vi "notasdealumnos.vi"() -> ()   [LabVIEW 2013]
panel:
  out "Sobresaliente":bool
  out "Muy bueno":bool
  out "Bueno":bool
  out "Reprobado":bool
  out "91-100 Sobresaliente":dbl
  out "81-90 Muy bueno":dbl
  out "60-80 Bueno":dbl
  out "1-59 Reprobado":dbl
  out "Notas":dbl
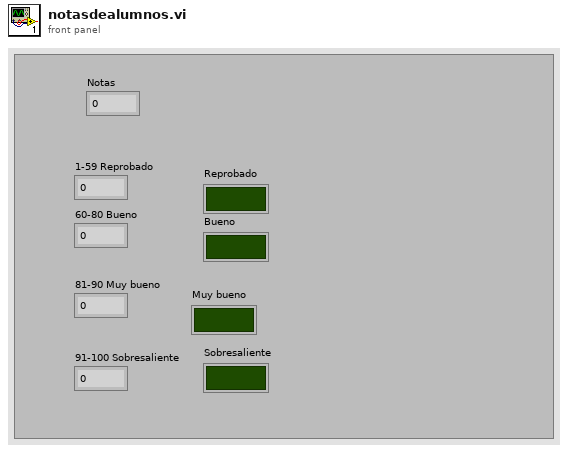
[diagram p1: front panel]
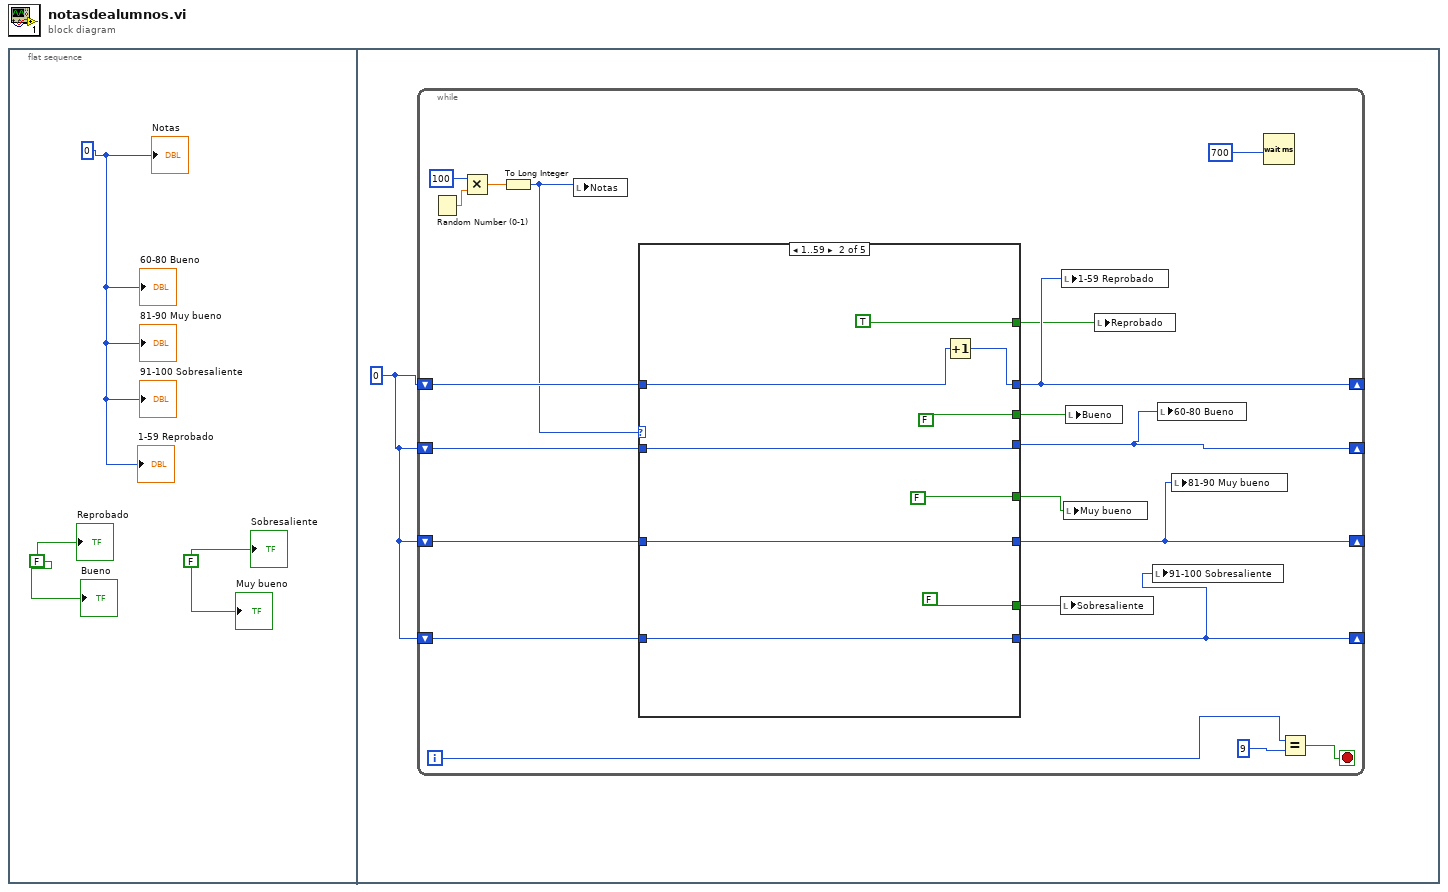
[diagram p0: block diagram]
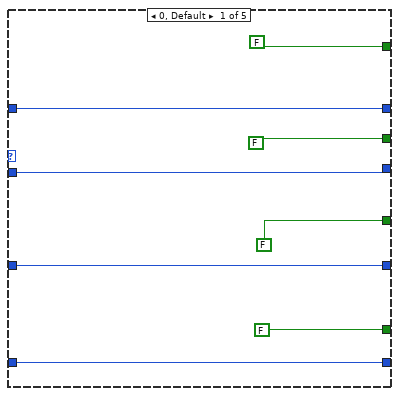
[diagram p2: hidden frame]
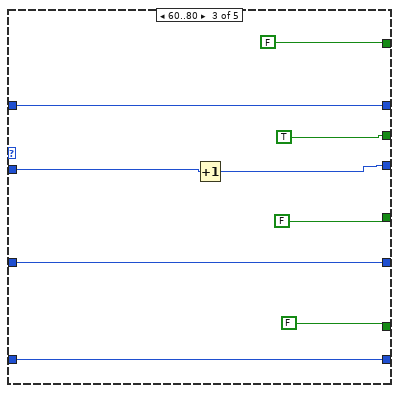
[diagram p3: hidden frame]
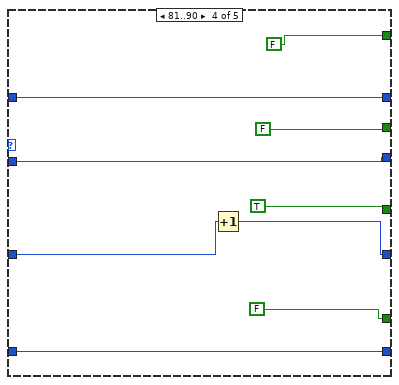
[diagram p4: hidden frame]
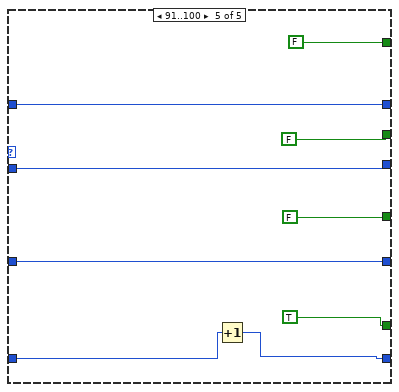
[diagram p5: hidden frame]
diagram:
  n1 = flat-sequence {
    frame #0 {
      w1 = FALSE
      w2 = FALSE
      w3 = 0
      "Notas" <- w3
      "1-59 Reprobado" <- w3
      "60-80 Bueno" <- w3
      "81-90 Muy bueno" <- w3
      "91-100 Sobresaliente" <- w3
      "Reprobado" <- w2
      "Bueno" <- w2
      "Muy bueno" <- w1
      "Sobresaliente" <- w1
    }
    frame #1 {
      w4 = 0
      n2 = while {
        shift-right: [w17] -> _
        shift-left: w4 -> [w21]
        shift-right: [w12] -> _
        shift-left: w4 -> [w20]
        shift-right: [w11] -> _
        shift-left: w4 -> [w19]
        shift-right: [w10] -> _
        shift-left: w4 -> [w18]
        i -> [w6]
        stop <- w9 stop-if-true
        n3 = Random Number (0-1)() -> (number: 0 to 1=w23:dbl)
        n4 = Multiply(x=100, y=w23) -> (x*y=w22:dbl)
        n5 = To Long Integer(number=w22) -> (32bit integer=w5:i32)
        n6 = local write "Notas"(w5) -> ()
        n7 = case shown="1..59" w5 {
          tunnel: w21 -> [w32 w38 w50 w59 w68]
          tunnel: w20 -> [w31 w41 w43 w58 w67]
          tunnel: w19 -> [w30 w40 w48 w52 w66]
          tunnel: w18 -> [w29 w39 w49 w57 w61]
          tunnel: [w32 w37 w50 w59 w68] -> w17
          tunnel: [w31 w41 w42 w58 w67] -> w12
          tunnel: [w30 w40 w48 w51 w66] -> w11
          tunnel: [w29 w39 w49 w57 w60] -> w10
          tunnel: [FALSE TRUE FALSE FALSE FALSE] -> w16
          tunnel: [FALSE FALSE TRUE FALSE FALSE] -> w15
          tunnel: [FALSE FALSE FALSE TRUE FALSE] -> w14
          tunnel: [FALSE FALSE FALSE FALSE TRUE] -> w13
          frame 0, Default {
          }
          frame 1..59 {
            n8 = Increment(x=w38) -> (x+1=w37:i32)
          }
          frame 60..80 {
            n9 = Increment(x=w43) -> (x+1=w42:i32)
          }
          frame 81..90 {
            n10 = Increment(x=w52) -> (x+1=w51:i32)
          }
          frame 91..100 {
            n11 = Increment(x=w61) -> (x+1=w60:i32)
          }
        }
        n12 = local write "Sobresaliente"(w13) -> ()
        n13 = local write "1-59 Reprobado"(w17) -> ()
        n14 = local write "Muy bueno"(w14) -> ()
        n15 = local write "Bueno"(w15) -> ()
        n16 = local write "Reprobado"(w16) -> ()
        n17 = local write "91-100 Sobresaliente"(w10) -> ()
        n18 = local write "60-80 Bueno"(w12) -> ()
        n19 = local write "81-90 Muy bueno"(w11) -> ()
        n20 = Wait (ms)(milliseconds to wait=700) -> ()  [unwired: 1 out]
        n21 = Equal?(x=w6, y=9) -> (x = y?=w9:bool)
      }
    }
  }
